vi "Library2.vi"(0 "Message_command_in":T1, 3 "error in (no error)":errorcluster) -> (7 "Message_command out":T1, 10 "error out":errorcluster)   [LabVIEW 2020]
uses:
  Command_Message.ctl
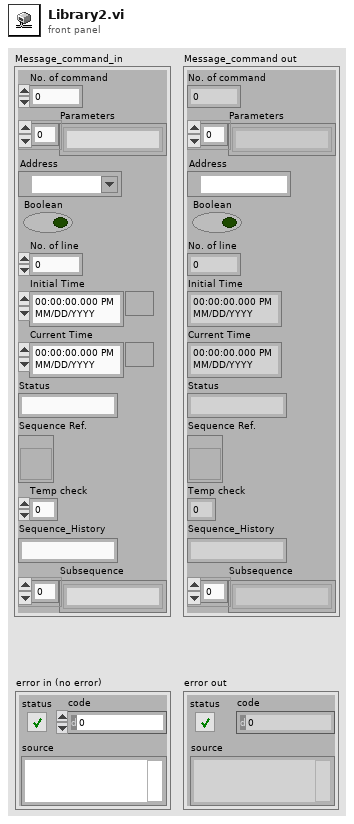
[diagram p1: front panel]
types:
  T1 = typedef "Command_Message.ctl" = cluster{"No. of command":i32, "Parameters":string[], "Address":refnum<visa-resource-name>, "Boolean":bool, "No. of line":i32, "Initial Time":timestamp, "Current Time":timestamp, "Status":string, "Sequence Ref.":refnum<vi>, "Temp check":i32, "Sequence_History":string, "Subsequence":string[]}
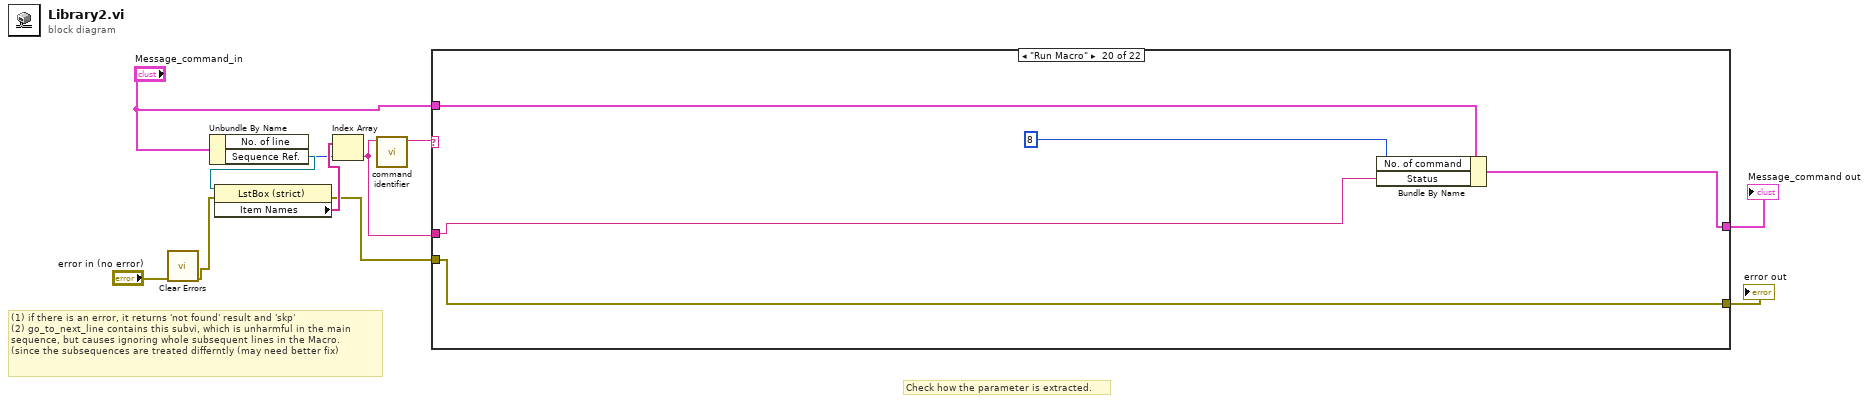
[diagram p0: block diagram]
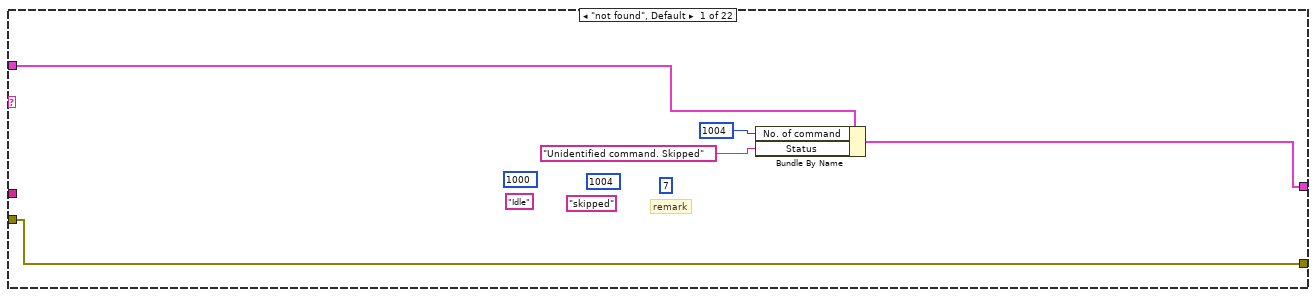
[diagram p2: hidden frame]
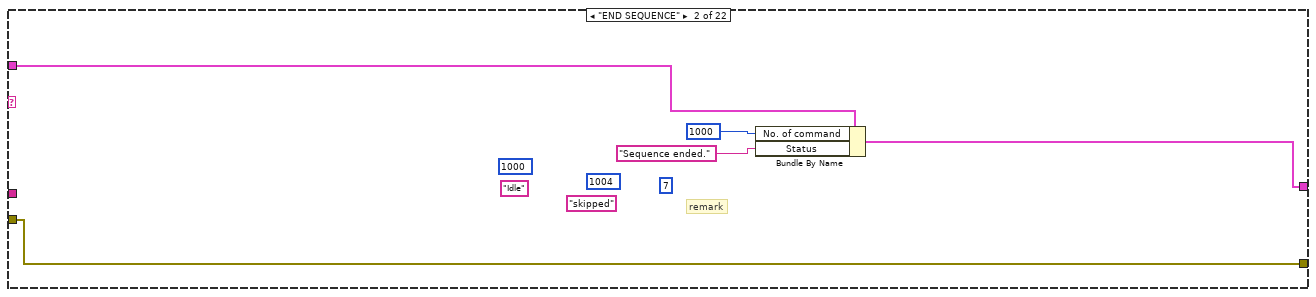
[diagram p3: hidden frame]
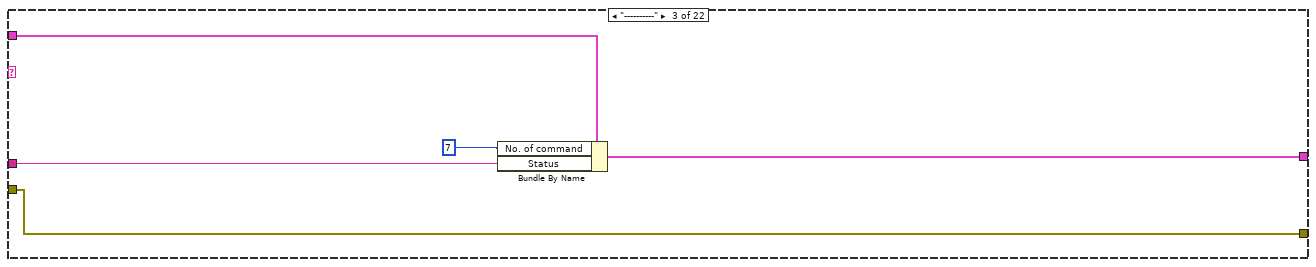
[diagram p4: hidden frame]
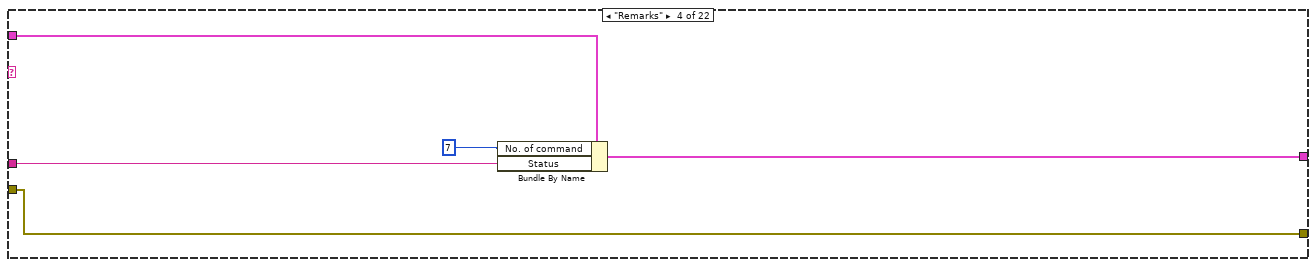
[diagram p5: hidden frame]
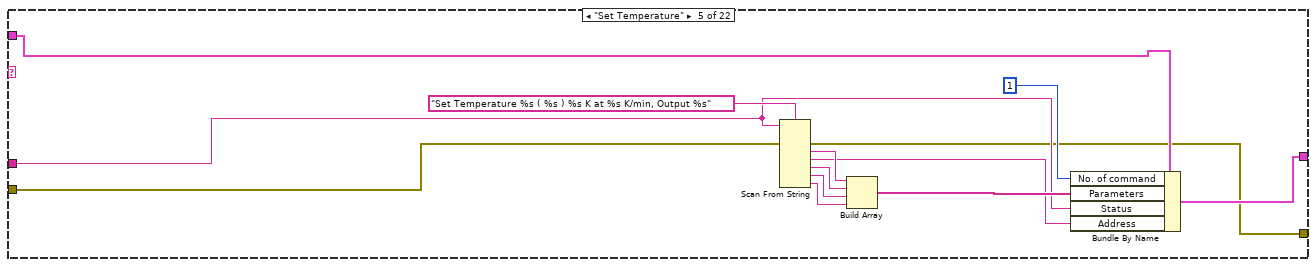
[diagram p6: hidden frame]
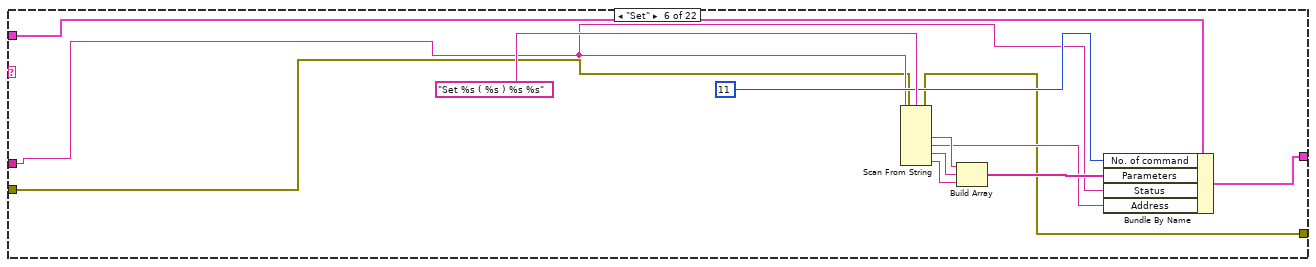
[diagram p7: hidden frame]
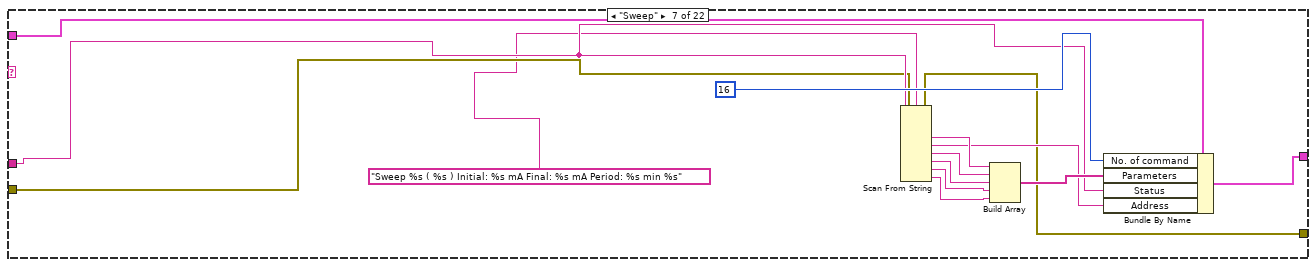
[diagram p8: hidden frame]
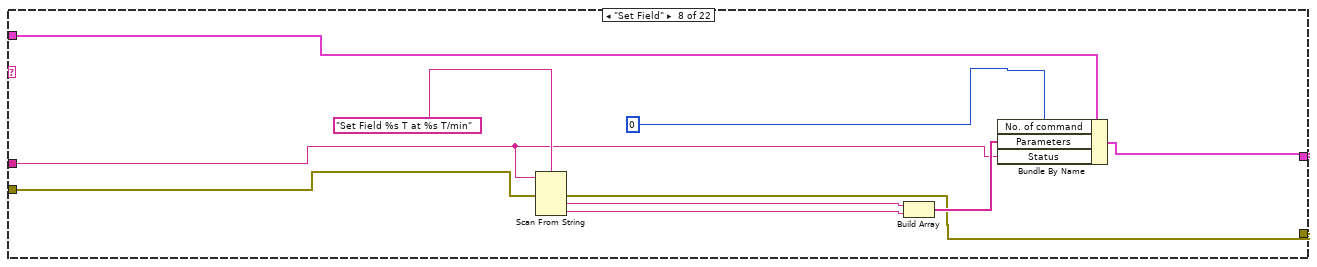
[diagram p9: hidden frame]
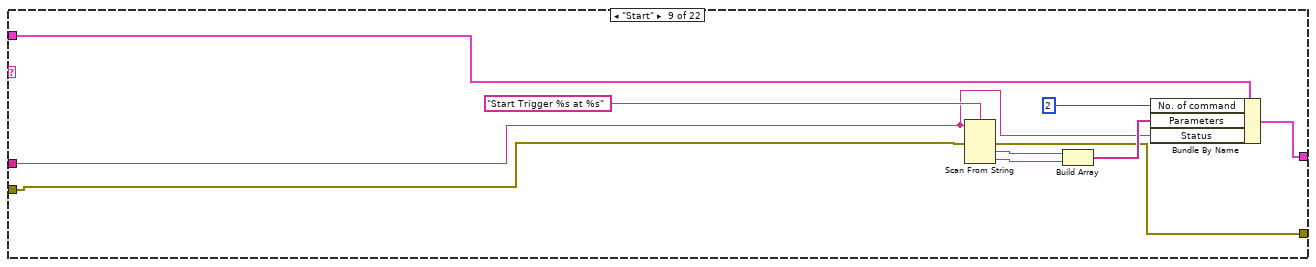
[diagram p10: hidden frame]
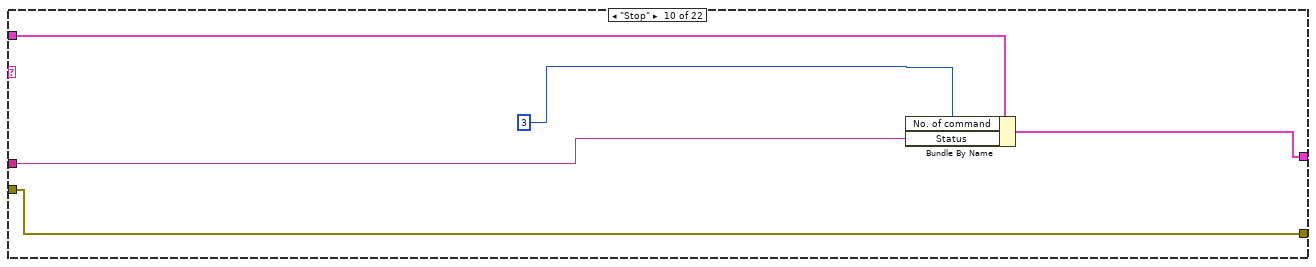
[diagram p11: hidden frame]
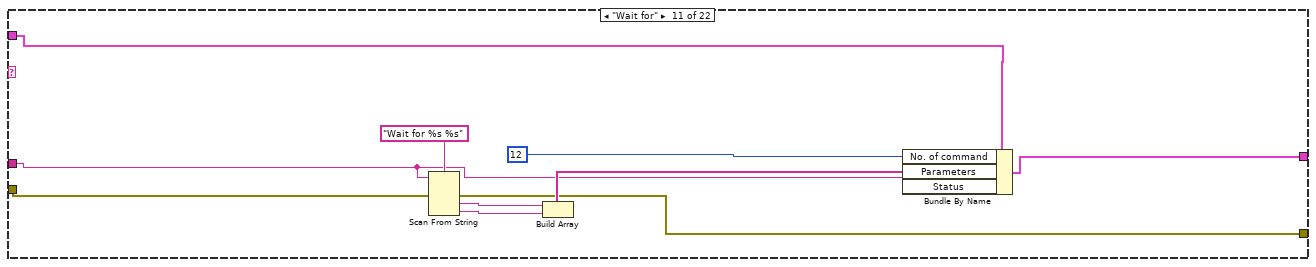
[diagram p12: hidden frame]
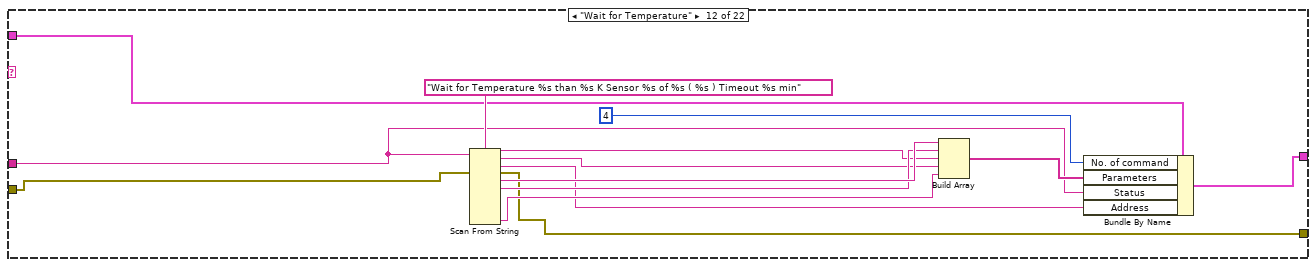
[diagram p13: hidden frame]
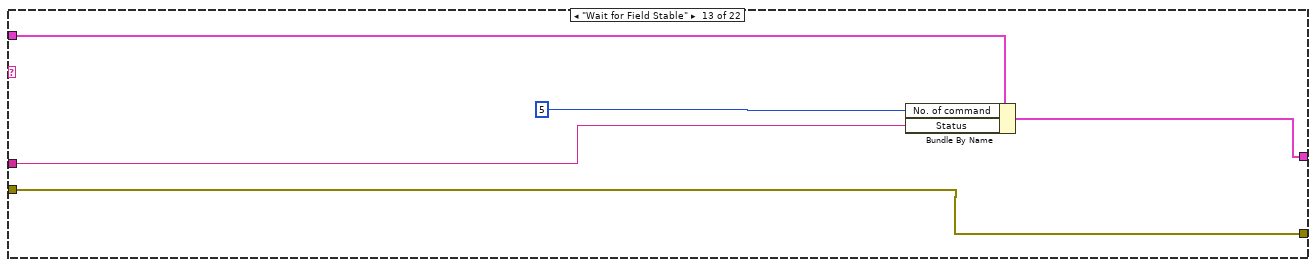
[diagram p14: hidden frame]
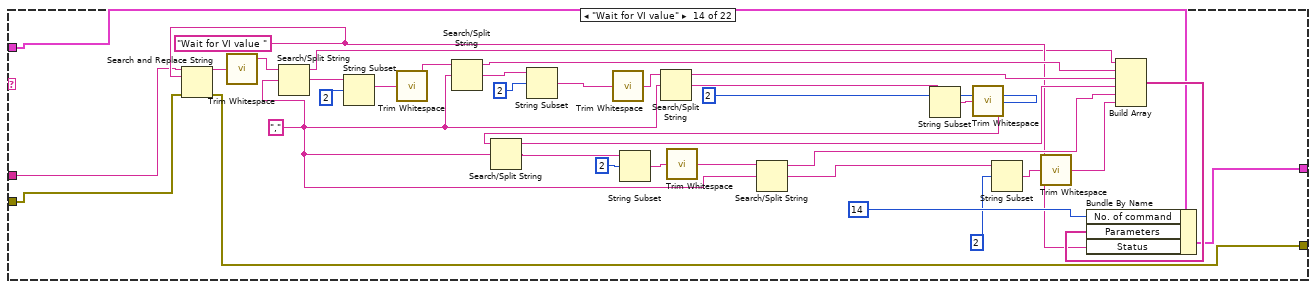
[diagram p15: hidden frame]
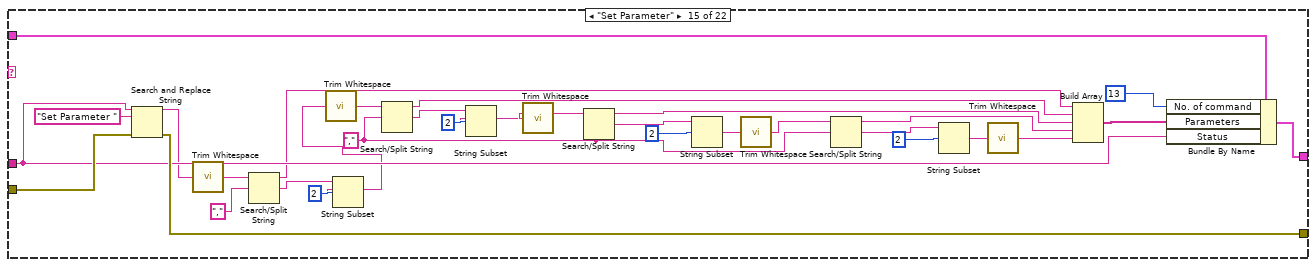
[diagram p16: hidden frame]
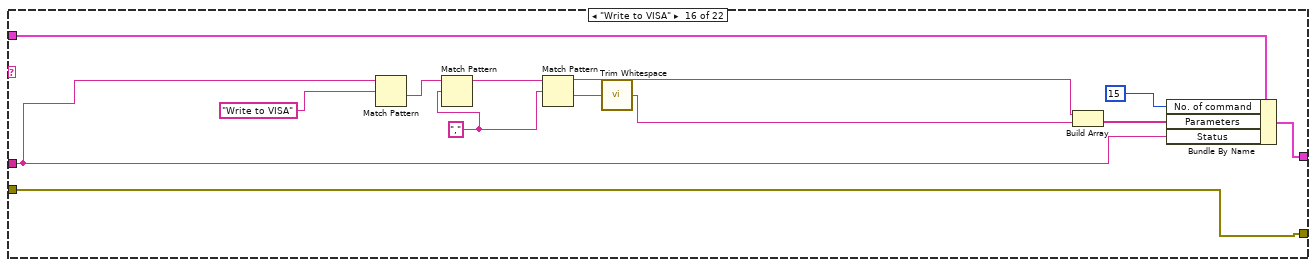
[diagram p17: hidden frame]
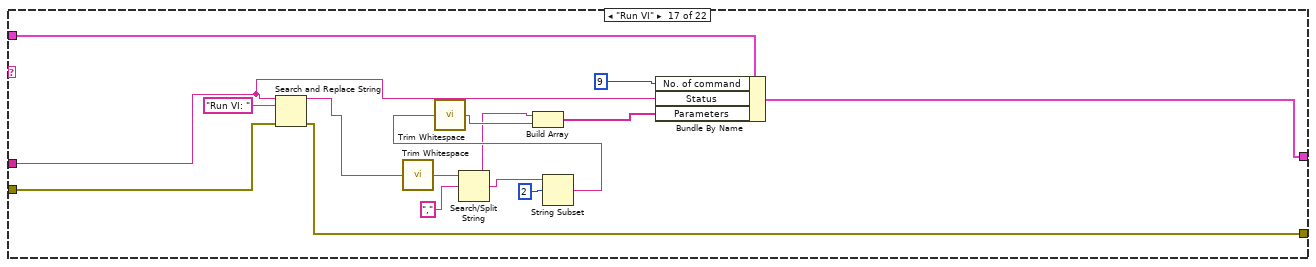
[diagram p18: hidden frame]
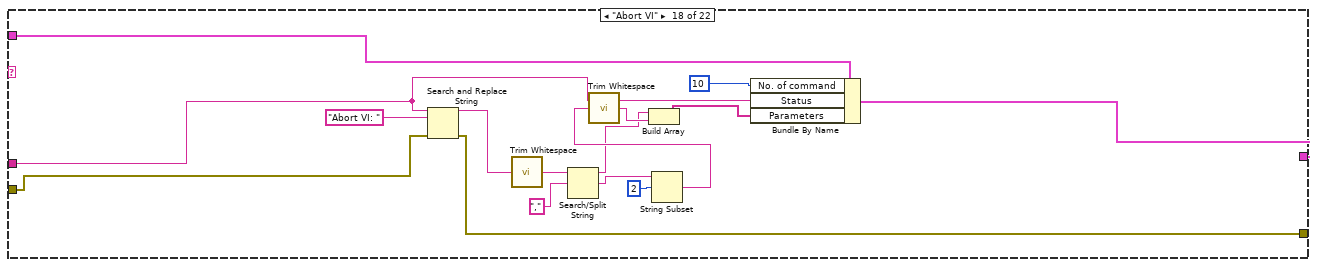
[diagram p19: hidden frame]
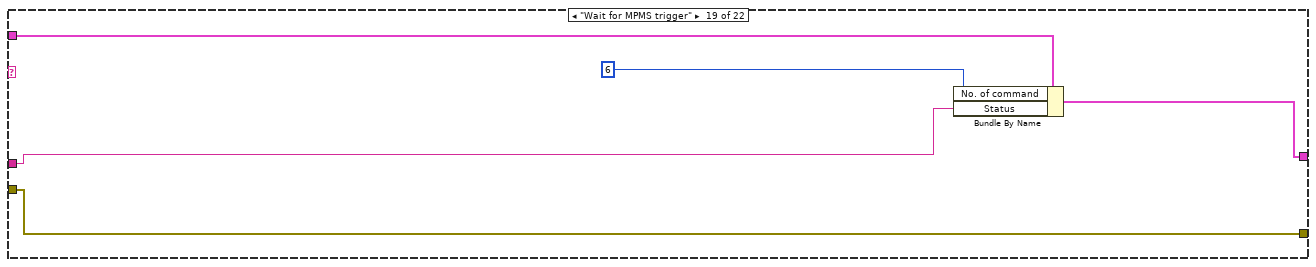
[diagram p20: hidden frame]
diagram:
  # "(1) if there is an error, it returns 'not found' result and 'skp'\n(2) go_to_next_line contains this subvi, which is unharmful in the main\nsequence, but causes ignoring whole subsequent lines in the Macro. \n(since the subsequences are treated differntly (may need better fix)"
  # "Check how the parameter is extracted."
  n1 = call <vilib>:"Clear Errors.vi"("error in (no error)"="error in (no error)") -> ("error out"=w1:errorcluster)  [unwired: 5 in, 1 out]
  n2 = Unbundle By Name("Message_command_in") -> ("No. of line"=w9:i32, "Sequence Ref."=w10:refnum<vi>)
  n3 = property on="Property Node" class="LstBox (strict)"(reference=w10, error in=w1) -> (error out=w5:errorcluster, "Item Names"=w11:string[])  [unwired: 1 out]
  n4 = Index Array(array=w11, index=w9) -> (element=w3:string)
  n5 = call "command identifier.vi"("Input command"=w3) -> ("Identifield command"=w8:string)  [unwired: 10 in]
  n6 = case shown="\"Run Macro\"" w8 {
    tunnel: w3 -> [_ _ w25 w30 w34 w48 w63 w73 w81 w91 w96 w109 w123 w135 w168 w197 w214 w232 w241 w246 w249 w254]
    tunnel: "Message_command_in" -> [w14 w19 w24 w29 w35 w49 w64 w75 w85 w93 w100 w110 w122 w136 w169 w203 w219 w233 w240 w245 w251 w256]
    tunnel: [w13 w18 w23 w28 w36 w46 w61 w72 w84 w92 w97 w106 w121 w132 w172 w204 w218 w234 w239 w244 w250 w255] -> w6
    tunnel: w5 -> [w12 w17 w22 w27 w33 w47 w62 w74 w83 w94 w99 w108 w120 w133 w170 w196 w216 w231 w238 w243 w248 w253]
    tunnel: [w12 w17 w22 w27 w32 w45 w60 w71 w82 w94 w98 w107 w120 w134 w171 w196 w215 w230 w238 w243 w248 w253] -> w4
    frame "not found", Default {
      (unwired) 7 ("No. of command")
      (unwired) "skipped" ("Status")
      (unwired) 1004 ("No. of command")
      (unwired) "Idle" ("Status")
      (unwired) 1000 ("No. of command")
      # "remark"
      n7 = Bundle By Name(cluster=w14, "No. of command"=1004, "Status"="Unidentified command. Skipped") -> (w13:T1)
    }
    frame "END SEQUENCE" {
      (unwired) 7 ("No. of command")
      (unwired) "skipped" ("Status")
      (unwired) 1004 ("No. of command")
      (unwired) "Idle" ("Status")
      (unwired) 1000 ("No. of command")
      # "remark"
      n8 = Bundle By Name(cluster=w19, "No. of command"=1000, "Status"="Sequence ended.") -> (w18:T1)
    }
    frame "----------" {
      n9 = Bundle By Name(cluster=w24, "No. of command"=7, "Status"=w25) -> (w23:T1)
    }
    frame "Remarks" {
      n10 = Bundle By Name(cluster=w29, "No. of command"=7, "Status"=w30) -> (w28:T1)
    }
    frame "Set Temperature" {
      n11 = Scan From String(format string="Set Temperature %s ( %s ) %s K at %s K/min, Output %s", input string=w34, error in=w33) -> (error out=w32:errorcluster, output 1=w43:string, output 2=w37:string, output 3=w42:string, output 4=w41:string, output 5=w40:string)  [unwired: 6 in, 2 out]
      n12 = Build Array(w43, w42, w41, w40) -> (w38:string[])
      n13 = Bundle By Name(cluster=w35, "No. of command"=1, "Parameters"=w38, "Status"=w34, "Address"=w37) -> (w36:T1)
    }
    frame "Set" {
      n14 = Scan From String(format string="Set %s ( %s ) %s %s", input string=w48, error in=w47) -> (error out=w45:errorcluster, output 1=w55:string, output 2=w50:string, output 3=w54:string, output 4=w53:string)  [unwired: 5 in, 2 out]
      n15 = Build Array(w55, w54, w53) -> (w52:string[])
      n16 = Bundle By Name(cluster=w49, "No. of command"=11, "Parameters"=w52, "Status"=w48, "Address"=w50) -> (w46:T1)
    }
    frame "Sweep" {
      n17 = Scan From String(format string="Sweep %s ( %s ) Initial: %s mA Final: %s mA Period: %s min %s", input string=w63, error in=w62) -> (error out=w60:errorcluster, output 1=w70:string, output 2=w65:string, output 3=w69:string, output 4=w68:string, output 5=w59:string, output 6=w58:string)  [unwired: 7 in, 2 out]
      n18 = Build Array(w70, w69, w68, w59, w58) -> (w67:string[])
      n19 = Bundle By Name(cluster=w64, "No. of command"=16, "Parameters"=w67, "Status"=w63, "Address"=w65) -> (w61:T1)
    }
    frame "Set Field" {
      n20 = Scan From String(format string="Set Field %s T at %s T/min", input string=w73, error in=w74) -> (error out=w71:errorcluster, output 1=w79:string, output 2=w78:string)  [unwired: 3 in, 2 out]
      n21 = Build Array(w79, w78) -> (w76:string[])
      n22 = Bundle By Name(cluster=w75, "No. of command"=0, "Parameters"=w76, "Status"=w73) -> (w72:T1)
    }
    frame "Start" {
      n23 = Scan From String(format string="Start Trigger %s at %s", input string=w81, error in=w83) -> (error out=w82:errorcluster, output 1=w89:string, output 2=w88:string)  [unwired: 3 in, 2 out]
      n24 = Build Array(w89, w88) -> (w87:string[])
      n25 = Bundle By Name(cluster=w85, "No. of command"=2, "Parameters"=w87, "Status"=w81) -> (w84:T1)
    }
    frame "Stop" {
      n26 = Bundle By Name(cluster=w93, "No. of command"=3, "Status"=w91) -> (w92:T1)
    }
    frame "Wait for" {
      n27 = Scan From String(format string="Wait for %s %s", input string=w96, error in=w99) -> (error out=w98:errorcluster, output 1=w104:string, output 2=w103:string)  [unwired: 3 in, 2 out]
      n28 = Build Array(w104, w103) -> (w101:string[])
      n29 = Bundle By Name(cluster=w100, "No. of command"=12, "Parameters"=w101, "Status"=w96) -> (w97:T1)
    }
    frame "Wait for Temperature" {
      n30 = Scan From String(format string="Wait for Temperature %s than %s K Sensor %s of %s ( %s ) Timeout %s min", input string=w109, error in=w108) -> (error out=w107:errorcluster, output 1=w117:string, output 2=w116:string, output 3=w115:string, output 4=w114:string, output 5=w112:string, output 6=w113:string)  [unwired: 7 in, 2 out]
      n31 = Build Array(w117, w116, w115, w114, w113) -> (w111:string[])
      n32 = Bundle By Name(cluster=w110, "No. of command"=4, "Parameters"=w111, "Status"=w109, "Address"=w112) -> (w106:T1)
    }
    frame "Wait for Field Stable" {
      n33 = Bundle By Name(cluster=w122, "No. of command"=5, "Status"=w123) -> (w121:T1)
    }
    frame "Wait for VI value" {
      w130 = "," ("search string/char (-)")
      w137 = "Wait for VI value " ("search string")
      n34 = Search and Replace String(input string=w135, search string=w137, error in=w133) -> (result string=w142:string, error out=w134:errorcluster)  [unwired: 5 in, 2 out]
      n35 = call <vilib>:"Trim Whitespace.vi"("string"=w142) -> ("trimmed string"=w131:string)  [unwired: 1 in]
      n36 = Search/Split String(string=w131, search string/char (-)=w130) -> (substring before match=w125:string, match + rest of string=w128:string)  [unwired: 1 in, 1 out]
      n37 = String Subset(string=w128, offset (0)=2) -> (substring=w127:string)  [unwired: 1 in]
      n38 = call <vilib>:"Trim Whitespace.vi"("string"=w127) -> ("trimmed string"=w126:string)  [unwired: 1 in]
      n39 = Search/Split String(string=w126, search string/char (-)=w130) -> (substring before match=w156:string, match + rest of string=w144:string)  [unwired: 1 in, 1 out]
      n40 = String Subset(string=w144, offset (0)=2) -> (substring=w145:string)  [unwired: 1 in]
      n41 = call <vilib>:"Trim Whitespace.vi"("string"=w145) -> ("trimmed string"=w140:string)  [unwired: 1 in]
      n42 = Search/Split String(string=w140, search string/char (-)=w130) -> (substring before match=w157:string, match + rest of string=w147:string)  [unwired: 1 in, 1 out]
      n43 = String Subset(string=w147, offset (0)=2) -> (substring=w148:string)  [unwired: 1 in]
      n44 = call <vilib>:"Trim Whitespace.vi"("string"=w148) -> ("trimmed string"=w141:string)  [unwired: 1 in]
      n45 = Search/Split String(string=w141, search string/char (-)=w130) -> (substring before match=w158:string, match + rest of string=w153:string)  [unwired: 1 in, 1 out]
      n46 = String Subset(string=w153, offset (0)=2) -> (substring=w152:string)  [unwired: 1 in]
      n47 = call <vilib>:"Trim Whitespace.vi"("string"=w152) -> ("trimmed string"=w154:string)  [unwired: 1 in]
      n48 = Search/Split String(string=w154, search string/char (-)=w130) -> (substring before match=w159:string, match + rest of string=w155:string)  [unwired: 1 in, 1 out]
      n49 = String Subset(string=w155, offset (0)=2) -> (substring=w150:string)  [unwired: 1 in]
      n50 = call <vilib>:"Trim Whitespace.vi"("string"=w150) -> ("trimmed string"=w138:string)  [unwired: 1 in]
      n51 = Build Array(w125, w156, w157, w158, w159, w138) -> (w139:string[])
      n52 = Bundle By Name(cluster=w136, "No. of command"=14, "Parameters"=w139, "Status"=w137) -> (w132:T1)
    }
    frame "Set Parameter" {
      w185 = "," ("search string/char (-)")
      n53 = Search and Replace String(input string=w168, search string="Set Parameter ", error in=w170) -> (result string=w163:string, error out=w171:errorcluster)  [unwired: 5 in, 2 out]
      n54 = call <vilib>:"Trim Whitespace.vi"("string"=w163) -> ("trimmed string"=w166:string)  [unwired: 1 in]
      n55 = Search/Split String(string=w166, search string/char (-)=",") -> (substring before match=w161:string, match + rest of string=w164:string)  [unwired: 1 in, 1 out]
      n56 = String Subset(string=w164, offset (0)=2) -> (substring=w162:string)  [unwired: 1 in]
      n57 = call <vilib>:"Trim Whitespace.vi"("string"=w162) -> ("trimmed string"=w182:string)  [unwired: 1 in]
      n58 = Search/Split String(string=w182, search string/char (-)=w185) -> (substring before match=w189:string, match + rest of string=w180:string)  [unwired: 1 in, 1 out]
      n59 = String Subset(string=w180, offset (0)=2) -> (substring=w179:string)  [unwired: 1 in]
      n60 = call <vilib>:"Trim Whitespace.vi"("string"=w179) -> ("trimmed string"=w188:string)  [unwired: 1 in]
      n61 = Search/Split String(string=w188, search string/char (-)=w185) -> (substring before match=w187:string, match + rest of string=w177:string)  [unwired: 1 in, 1 out]
      n62 = String Subset(string=w177, offset (0)=2) -> (substring=w176:string)  [unwired: 1 in]
      n63 = call <vilib>:"Trim Whitespace.vi"("string"=w176) -> ("trimmed string"=w186:string)  [unwired: 1 in]
      n64 = Search/Split String(string=w186, search string/char (-)=w185) -> (substring before match=w184:string, match + rest of string=w174:string)  [unwired: 1 in, 1 out]
      n65 = String Subset(string=w174, offset (0)=2) -> (substring=w173:string)  [unwired: 1 in]
      n66 = call <vilib>:"Trim Whitespace.vi"("string"=w173) -> ("trimmed string"=w183:string)  [unwired: 1 in]
      n67 = Build Array(w161, w189, w187, w184, w183) -> (w192:string[])
      n68 = Bundle By Name(cluster=w169, "No. of command"=13, "Parameters"=w192, "Status"=w168) -> (w172:T1)
    }
    frame "Write to VISA" {
      w199 = "," ("search string/char (-)")
      n69 = Match Pattern(string=w197, regular expression="Write to VISA" ("search string")) -> (after substring=w200:string)  [unwired: 1 in, 3 out]
      n70 = Match Pattern(string=w200, regular expression=w199) -> (after substring=w201:string)  [unwired: 1 in, 3 out]
      n71 = Match Pattern(string=w201, regular expression=w199) -> (before substring=w195:string, after substring=w202:string)  [unwired: 1 in, 2 out]
      n72 = call <vilib>:"Trim Whitespace.vi"("string"=w202) -> ("trimmed string"=w194:string)  [unwired: 1 in]
      n73 = Build Array(w195, w194) -> (w193:string[])
      n74 = Bundle By Name(cluster=w203, "No. of command"=15, "Parameters"=w193, "Status"=w197) -> (w204:T1)
    }
    frame "Run VI" {
      n75 = Search and Replace String(input string=w214, search string="Run VI: ", error in=w216) -> (result string=w209:string, error out=w215:errorcluster)  [unwired: 5 in, 2 out]
      n76 = call <vilib>:"Trim Whitespace.vi"("string"=w209) -> ("trimmed string"=w212:string)  [unwired: 1 in]
      n77 = Search/Split String(string=w212, search string/char (-)=",") -> (substring before match=w206:string, match + rest of string=w210:string)  [unwired: 1 in, 1 out]
      n78 = String Subset(string=w210, offset (0)=2) -> (substring=w208:string)  [unwired: 1 in]
      n79 = call <vilib>:"Trim Whitespace.vi"("string"=w208) -> ("trimmed string"=w207:string)  [unwired: 1 in]
      n80 = Build Array(w206, w207) -> (w220:string[])
      n81 = Bundle By Name(cluster=w219, "No. of command"=9, "Status"=w214, "Parameters"=w220) -> (w218:T1)
    }
    frame "Abort VI" {
      n82 = Search and Replace String(input string=w232, search string="Abort VI: " ("format string"), error in=w231) -> (result string=w225:string, error out=w230:errorcluster)  [unwired: 5 in, 2 out]
      n83 = call <vilib>:"Trim Whitespace.vi"("string"=w225) -> ("trimmed string"=w228:string)  [unwired: 1 in]
      n84 = Search/Split String(string=w228, search string/char (-)=",") -> (substring before match=w222:string, match + rest of string=w226:string)  [unwired: 1 in, 1 out]
      n85 = String Subset(string=w226, offset (0)=2) -> (substring=w224:string)  [unwired: 1 in]
      n86 = call <vilib>:"Trim Whitespace.vi"("string"=w224) -> ("trimmed string"=w223:string)  [unwired: 1 in]
      n87 = Build Array(w222, w223) -> (w236:string[])
      n88 = Bundle By Name(cluster=w233, "No. of command"=10, "Status"=w232, "Parameters"=w236) -> (w234:T1)
    }
    frame "Wait for MPMS trigger" {
      n89 = Bundle By Name(cluster=w240, "No. of command"=6, "Status"=w241) -> (w239:T1)
    }
    frame "Run Macro" {
      n90 = Bundle By Name(cluster=w245, "No. of command"=8, "Status"=w246) -> (w244:T1)
    }
    frame "END SUBsequence" {
      n91 = Bundle By Name(cluster=w251, "No. of command"=1007, "Status"=w249) -> (w250:T1)
    }
    frame "SubMacro" {
      n92 = Bundle By Name(cluster=w256, "No. of command"=1008, "Status"=w254) -> (w255:T1)
    }
  }
  "error out" <- w4
  "Message_command out" <- w6
